vi "security key.vi"() -> ()   [LabVIEW 2016]
panel:
  out "ALARM":bool
  out "DOOR":bool
  out "door open ?":bool
  out "inputted data crypted":string
  out "?":bool[](array[boolean])
  out "input character":string
  in  "stop":bool
  in  "VISA resource name":refnum<visa-resource-name>
  # "check the data"
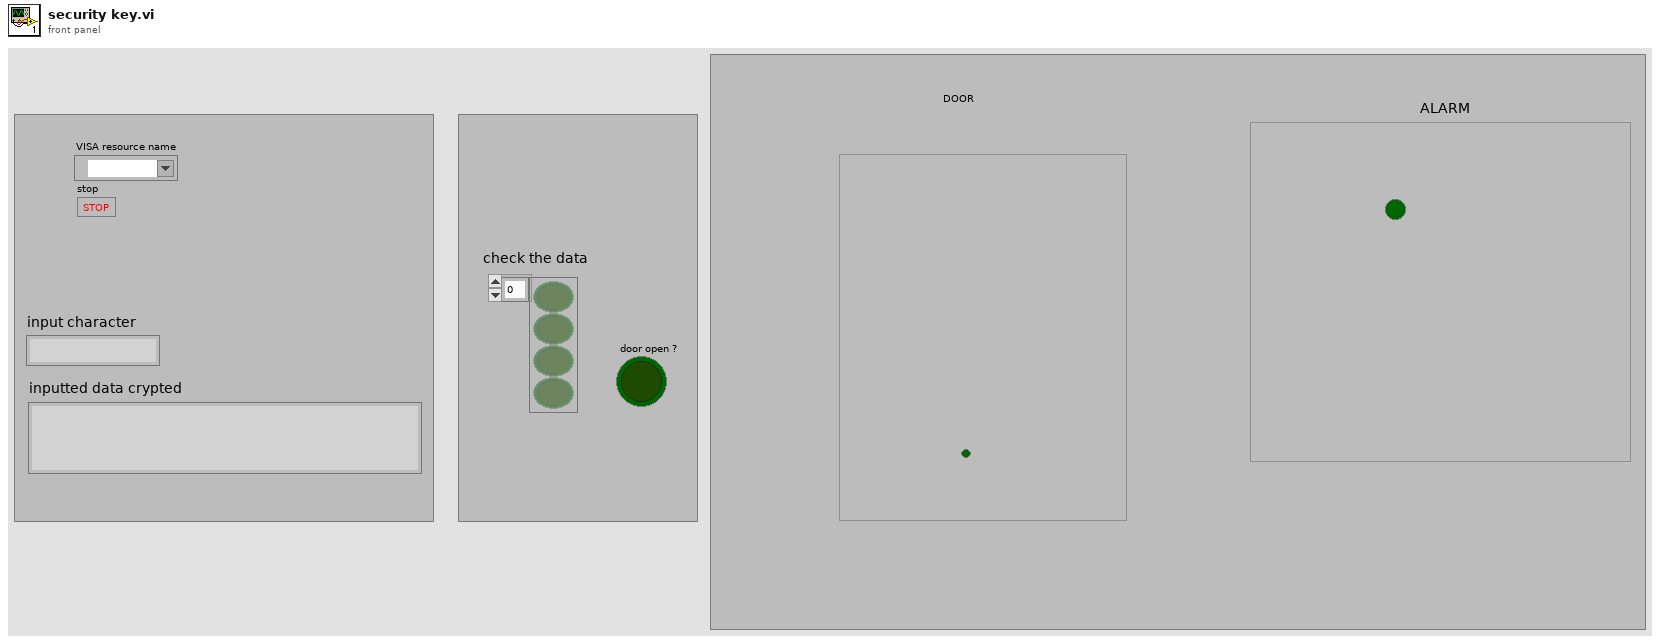
[diagram p1: front panel]
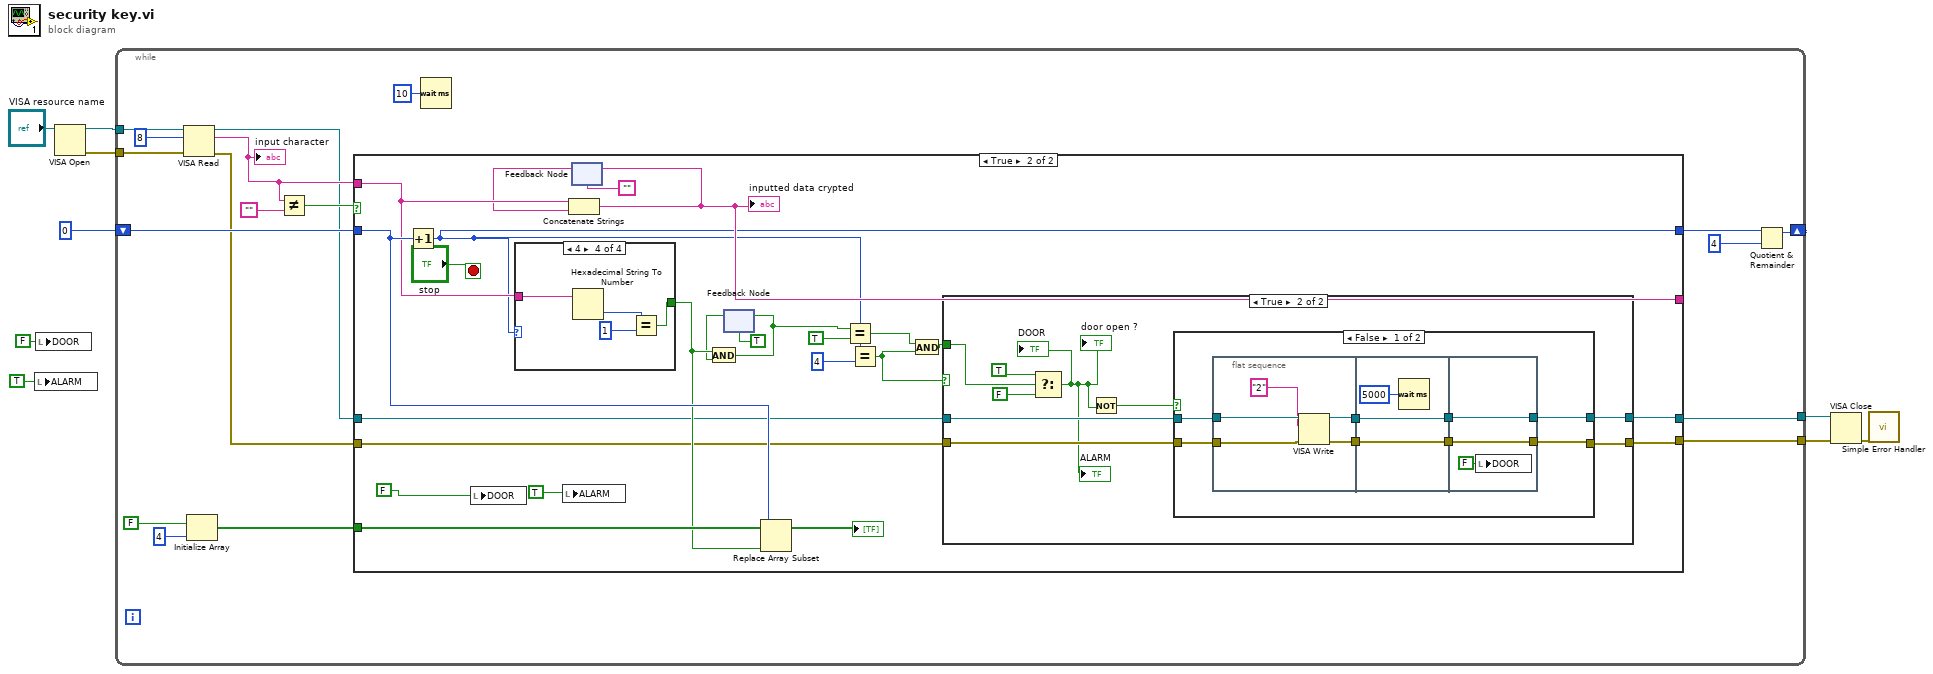
[diagram p0: block diagram]
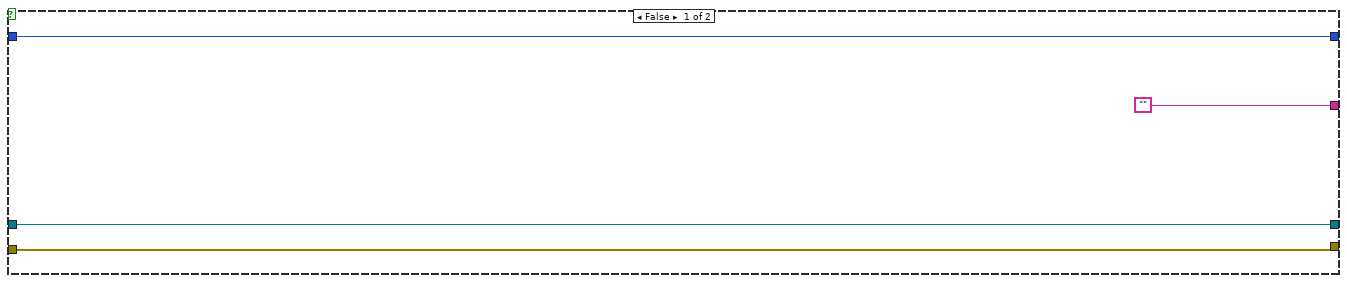
[diagram p2: hidden frame]
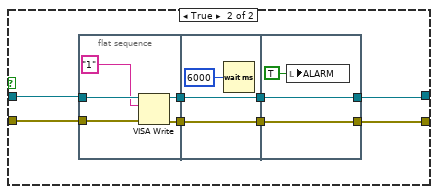
[diagram p4: hidden frame]
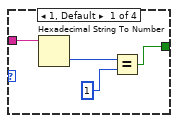
[diagram p5: hidden frame]
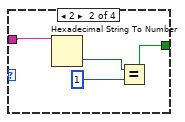
[diagram p6: hidden frame]
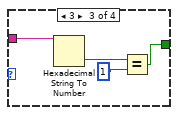
[diagram p7: hidden frame]
diagram:
  n1 = local write "ALARM"(TRUE ("Boolean")) -> ()
  n2 = local write "DOOR"(FALSE ("door")) -> ()
  n3 = VISA Open(VISA resource name="VISA resource name") -> (VISA resource name=w9:refnum<visa-resource-name>, error out=w8:errorcluster)  [unwired: 4 in]
  n4 = while {
    tunnel: w9 -> [w28]
    tunnel: w8 -> [w27]
    shift-right: [w18] -> _
    shift-left: 0 -> [w23]
    tunnel: [w11] -> w4
    tunnel: [w10] -> w3
    stop <- "stop" stop-if-true
    n5 = VISA Read(VISA resource name=w28, byte count=u32 8, error in (no error)=w27) -> (VISA resource name out=w13:refnum<visa-resource-name>, read buffer=w19:string, error out=w12:errorcluster)  [unwired: 1 out]
    "input character" <- w19
    n6 = Initialize Array(FALSE, 4 ("dimension size")) -> (w14:bool[])
    n7 = Not Equal?(x=w19, y="") -> (x != y?=w24:bool)
    n8 = case shown="True" w24 {
      tunnel: w23 -> [w32 w55]
      tunnel: [w32 w45] -> w22
      tunnel: w19 -> [_ w53]
      tunnel: ["" w51] -> _
      tunnel: w14 -> [_ w49]
      tunnel: w13 -> [w30 w39]
      tunnel: w12 -> [w29 w38]
      tunnel: [w30 w37] -> w11
      tunnel: [w29 w36] -> w10
      frame False {
      }
      frame True {
        n9 = Increment(x=w55) -> (x+1=w45:i32)
        n10 = local write "DOOR"(FALSE) -> ()
        n11 = case shown="4" w45 {
          tunnel: w53 -> [w107 w111 w115 w119]
          tunnel: [w108 w112 w116 w120] -> w47
          frame 1, Default {
            n12 = Hexadecimal String To Number(string=w107) -> (number=w106:u32)  [unwired: 2 in, 1 out]
            n13 = Equal?(x=w106, y=u32 1) -> (x = y?=w108:bool)
          }
          frame 2 {
            n14 = Hexadecimal String To Number(string=w111) -> (number=w110:u32)  [unwired: 2 in, 1 out]
            n15 = Equal?(x=w110, y=u32 1) -> (x = y?=w112:bool)
          }
          frame 3 {
            n16 = Hexadecimal String To Number(string=w115) -> (number=w114:u32)  [unwired: 2 in, 1 out]
            n17 = Equal?(x=w114, y=u32 1) -> (x = y?=w116:bool)
          }
          frame 4 {
            n18 = Hexadecimal String To Number(string=w119) -> (number=w118:u32)  [unwired: 2 in, 1 out]
            n19 = Equal?(x=w118, y=u32 1) -> (x = y?=w120:bool)
          }
        }
        n20 = local write "ALARM"(TRUE) -> ()
        n21 = feedback #1("") -> (w52:string)
        n22 = Concatenate Strings(w53, w52) -> (w51:string)
        "inputted data crypted" <- w51
        n23 = feedback-in #1(w51) -> ()
        n24 = feedback #2(TRUE) -> (w46:bool)
        n25 = And(x=w47, y=w46) -> (x .and. y?=w43:bool)
        n26 = feedback-in #2(w43) -> ()
        n27 = Replace Array Subset(array=w49, new element=w47, index=w55) -> (→"?":bool[])
        n28 = Equal?(x=w43, y=TRUE) -> (x = y?=w41:bool)
        n29 = Equal?(x=w45, y=4) -> (x = y?=w35:bool)
        n30 = And(x=w41, y=w35) -> (x .and. y?=w40:bool)
        n31 = case shown="True" w35 {
          tunnel: w40 -> [_ w66]
          tunnel: w39 -> [w57 w63]
          tunnel: w38 -> [w56 w62]
          tunnel: [w57 w61] -> w37
          tunnel: [w56 w60] -> w36
          frame False {
          }
          frame True {
            n32 = Select(t=TRUE, s=w66, f=FALSE) -> (s? t:f=w58:bool)
            "door open ?" <- w58
            "DOOR" <- w58
            "ALARM" <- w58
            n33 = Not(x=w58) -> (.not. x?=w59:bool)
            n34 = case shown="False" w59 {
              tunnel: w63 -> [w74 w93]
              tunnel: w62 -> [w73 w92]
              tunnel: [w72 w89] -> w61
              tunnel: [w71 w88] -> w60
              frame False {
                n35 = flat-sequence {
                  tunnel: w74 -> [w79]
                  tunnel: w73 -> [w78]
                  tunnel: [w77] -> w70
                  tunnel: [w76] -> w69
                  tunnel: w70 -> [w82]
                  tunnel: w69 -> [w81]
                  tunnel: [w82] -> w68
                  tunnel: [w81] -> w67
                  tunnel: [w84] -> w71
                  tunnel: [w85] -> w72
                  tunnel: w68 -> [w85]
                  tunnel: w67 -> [w84]
                  frame #0 {
                    n36 = VISA Write(VISA resource name=w79, write buffer="2", error in (no error)=w78) -> (VISA resource name out=w77:refnum<visa-resource-name>, error out=w76:errorcluster)  [unwired: 1 out]
                  }
                  frame #1 {
                    n37 = Wait (ms)(milliseconds to wait=u32 5000) -> ()  [unwired: 1 out]
                  }
                  frame #2 {
                    n38 = local write "DOOR"(FALSE ("door")) -> ()
                  }
                }
              }
              frame True {
                n39 = flat-sequence {
                  tunnel: w93 -> [w98]
                  tunnel: w92 -> [w97]
                  tunnel: [w95] -> w91
                  tunnel: [w94] -> w90
                  tunnel: w91 -> [w100]
                  tunnel: w90 -> [w99]
                  tunnel: [w100] -> w87
                  tunnel: [w99] -> w86
                  tunnel: [w103] -> w88
                  tunnel: [w104] -> w89
                  tunnel: w87 -> [w104]
                  tunnel: w86 -> [w103]
                  frame #0 {
                    n40 = VISA Write(VISA resource name=w98, write buffer="1", error in (no error)=w97) -> (VISA resource name out=w95:refnum<visa-resource-name>, error out=w94:errorcluster)  [unwired: 1 out]
                  }
                  frame #1 {
                    n41 = Wait (ms)(milliseconds to wait=u32 6000) -> ()  [unwired: 1 out]
                  }
                  frame #2 {
                    n42 = local write "ALARM"(TRUE ("Boolean")) -> ()
                  }
                }
              }
            }
          }
        }
      }
    }
    n43 = Wait (ms)(milliseconds to wait=u32 10) -> ()  [unwired: 1 out]
    n44 = Quotient & Remainder(x=w22, y=4) -> (x-y*floor(x/y)=w18:i32)  [unwired: 1 out]
  }
  n45 = VISA Close(VISA resource name=w4, error in (no error)=w3) -> (error out=w6:errorcluster)
  n46 = call <vilib>:"Simple Error Handler.vi"("error in (no error)"=w6) -> ()  [unwired: 4 in, 5 out]
